vi "lab3.vi"() -> ()   [LabVIEW 2019]
uses:
  <vilib>/imath/engines/lvmath2/RunTimeEngine/BuiltInFunctions/iir_elliptic/NIMS_[2o]_iir_elliptic(I32,DBL2,V,Str).vi
  <vilib>/imath/engines/lvmath2/RunTimeEngine/ErrorHandling/NIMS_Create Error From Enums.vi
  <vilib>/imath/engines/lvmath/Plug In/Control Design/BuiltInFunctions/tf/NIMS_CD_tf(num,den,Ts).vi
  <vilib>/imath/engines/lvmath2/RunTimeEngine/BuiltInFunctions/iir_elliptic/NIMS_[3o]_iir_elliptic(I32,DBL2,V,Str).vi
  <vilib>/imath/engines/lvmath/Plug In/Control Design/BuiltInFunctions/zpk/NIMS_CD_zpk(zeros,poles,k,Ts).vi
  <vilib>/imathl/engines/lvmath/Functions/Error Handling/Create Error.vi
  <vilib>/imath/engines/lvmath2/RunTimeEngine/BuiltInFunctions/iir_elliptic/NIMS_[4o]_iir_elliptic(I32,DBL2,V,Str).vi
  <vilib>/imath/engines/lvmath/Plug In/Control Design/BuiltInFunctions/ss/NIMS_CD_ss(A,B,C,D).vi
  <vilib>/imath/engines/lvmath2/RunTimeEngine/NodeEndStatement/NIMS_NodeEndStatement_Output.vi
  <instcachedir>/0/NIMS_NodeEndStatement_Output_53EC0D466D134D7ABD903AC30B43404B.lvgen/NIMS_NodeEndStatement_Output_53EC0D466D134D7ABD903AC30B43404B_011.vi
  <instcachedir>/0/NIMS_NodeEndStatement_Output_53EC0D466D134D7ABD903AC30B43404B.lvgen/NIMS_NodeEndStatement_Output_53EC0D466D134D7ABD903AC30B43404B_010.vi
  <instcachedir>/0/NIMS_NodeEndStatement_Output_53EC0D466D134D7ABD903AC30B43404B.lvgen/NIMS_NodeEndStatement_Output_53EC0D466D134D7ABD903AC30B43404B_009.vi
  <vilib>/imath/engines/lvmath2/RunTimeEngine/ErrorHandling/NIMS_Finalize Error.vi
  <vilib>/addons/Control Design/_Time Response Analysis/Time Response.llb/Time Response subVI/cd_Step Response (State-Space).vi
  <vilib>/addons/Control Design/_Frequency Response Analysis/Frequency Response.llb/Frequency Response subVI/cd_Bode (State Space).vi
  <vilib>/addons/Control Design/_Utility/Model Viewer.llb/Model Viewer SubVI/cd_Draw State-Space Equation (SS).vi
  <vilib>/addons/Control Design/_Frequency Response Analysis/Frequency Response.llb/Frequency Response subVI/cd_Bode (Zero-Pole-Gain).vi
  <vilib>/addons/Control Design/_Time Response Analysis/Time Response.llb/Time Response subVI/cd_Step Response (Zero-Pole-Gain).vi
  <vilib>/addons/Control Design/_Utility/Model Viewer.llb/Model Viewer SubVI/cd_Draw Zero-Pole-Gain Equation (ZPK).vi
  <vilib>/addons/Control Design/_Frequency Response Analysis/Frequency Response.llb/Frequency Response subVI/cd_Bode (Transfer Function).vi
  <vilib>/addons/Control Design/_Time Response Analysis/Time Response.llb/Time Response subVI/cd_Step Response (Transfer Function).vi
  <vilib>/addons/Control Design/_Utility/Model Viewer.llb/Model Viewer SubVI/cd_Draw Transfer Function Equation (TF).vi
  <vilib>/addons/Control Design/_Utility/NI_CD_Model Viewer.lvlib
  <vilib>/addons/Control Design/_Time Response Analysis/NI_CD_Time Response.lvlib
  <vilib>/addons/Control Design/_Frequency Response Analysis/NI_CD_Frequency Response.lvlib
panel:
  out "ФЧХ":cluster{"time":dbl[], dbl[]}[](graph)
  out "Нули, полюса и коэффициент усиления (zpk)":picture
  out "Реакция на ступенчатое воздействие":cluster{"time":dbl[], dbl[]}[](graph)=[{"time"=[0.0, 0.01, 0.02, 0.03, 0.04, 0.05, 0.06, 0.07, 0.08, 0.09, 0.1, 0.11, 0.12, 0.13, 0.14, 0.15, 0.16, 0.17, 0.18, 0.19, 0.2, 0.21, 0.22, 0.23, 0.24, 0.25, 0.26, 0.27, 0.28, 0.29, 0.3, 0.31, 0.32, 0.33, 0.34, 0.35000000000000003, 0.36, 0.37, 0.38, 0.39, 0.4, 0.41000000000000003, 0.42, 0.43, 0.44, 0.45, 0.46, 0.47000000000000003, 0.48, 0.49, 0.5, 0.51, 0.52, 0.53, 0.54, 0.55, 0.56, 0.5700000000000001, 0.58, 0.59, 0.6, 0.61, 0.62, 0.63, 0.64, 0.65, 0.66, 0.67, 0.68, 0.6900000000000001, 0.7000000000000001, 0.71, 0.72, 0.73, 0.74, 0.75, 0.76, 0.77, 0.78, 0.79, 0.8, 0.81, 0.8200000000000001, 0.8300000000000001, 0.84, 0.85, 0.86, 0.87, 0.88, 0.89, 0.9, 0.91, 0.92, 0.93, 0.9400000000000001, 0.9500000000000001, 0.96, 0.97, 0.98, 0.99, 1.0], [0.0, 3.6082865061234616e-06, 1.1407278521072656e-05, 2.9529784958030634e-05, 6.642330456811847e-05, 0.00013503170249437238, 0.0002548548609154596, 0.0004541695796313746, 0.0007725569985214442, 0.0012637784461943145, 0.0019989621543555023, 0.003069999296471257, 0.004592993460926125, 0.006711559663559145, 0.009599726404238182, 0.013464158128184637, 0.018545388338242815, 0.025117739083195107, 0.03348760461422225, 0.04398979952247976, 0.05698171784936523, 0.07283512155630463, 0.09192547485599553, 0.11461886387244882, 0.14125668546765777, 0.17213844925750407, 0.20750320518044707, 0.2475102759907256, 0.29222012880100523, 0.34157635049365703, 0.3953897864575091, 0.4533259492913405, 0.5148967939113728, 0.579457880307616, 0.6462118005760611, 0.7142185322522965, 0.7824130992479892, 0.8496305834265399, 0.9146381473654828, 0.9761733198830131, 1.0329873819716318, 1.083892296189833, 1.1278092731232305, 1.1638167900206793, 1.191195693197778, 1.2094689478589153, 1.2184336620214729, 1.2181832139346669, 1.2091176555606453, 1.191941040408115, 1.1676449153653718, 1.1374778975653794, 1.1029019953315176, 1.0655370872304384, 1.0270957013066055, 0.9893108920932084, 0.9538605515110161, 0.9222918708899738, 0.8959498617110293, 0.8759138185733986, 0.8629453575615864, 0.8574511882916371, 0.8594630943828092, 0.8686367349695323, 0.8842698822165649, 0.9053396306961685, 0.9305570161479116, 0.9584364302320009, 0.987376281517763, 1.0157465941619432, 1.041978709252556, 1.0646520019267478, 1.0825725766873904, 1.0948392620397485, 1.1008928822866797, 1.1005457078265957, 1.0939891258287846, 1.0817788649680364, 1.0647984729633668, 1.0442030983895345, 1.0213468811312547, 0.9976983250429551, 0.9747488376536154, 0.9539201158763563, 0.9364761935847676, 0.9234457298339228, 0.9155595125950468, 0.9132072149517516, 0.9164162242253882, 0.9248539457574722, 0.9378534532892434, 0.9544608181330321, 0.9735010039080574, 0.993657960958816, 1.0135635844875825, 1.031889581311644, 1.0474360710593627, 1.0592109474021638, 1.0664946358591876, 1.0688858688517833, 1.0663253920793205]}, {"time"=[0.0, 0.01, 0.02, 0.03, 0.04, 0.05, 0.06, 0.07, 0.08, 0.09, 0.1, 0.11, 0.12, 0.13, 0.14, 0.15, 0.16, 0.17, 0.18, 0.19, 0.2, 0.21, 0.22, 0.23, 0.24, 0.25, 0.26, 0.27, 0.28, 0.29, 0.3, 0.31, 0.32, 0.33, 0.34, 0.35000000000000003, 0.36, 0.37, 0.38, 0.39, 0.4, 0.41000000000000003, 0.42, 0.43, 0.44, 0.45, 0.46, 0.47000000000000003, 0.48, 0.49, 0.5, 0.51, 0.52, 0.53, 0.54, 0.55, 0.56, 0.5700000000000001, 0.58, 0.59, 0.6, 0.61, 0.62, 0.63, 0.64, 0.65, 0.66, 0.67, 0.68, 0.6900000000000001, 0.7000000000000001, 0.71, 0.72, 0.73, 0.74, 0.75, 0.76, 0.77, 0.78, 0.79, 0.8, 0.81, 0.8200000000000001, 0.8300000000000001, 0.84, 0.85, 0.86, 0.87, 0.88, 0.89, 0.9, 0.91, 0.92, 0.93, 0.9400000000000001, 0.9500000000000001, 0.96, 0.97, 0.98, 0.99, 1.0], [0.0, 3.470187299156327e-24, 4.370315472509466e-19, 4.1169111270240676e-16, 5.210188934862779e-14, 2.1899713849440105e-12, 4.575063221464954e-11, 5.889795375843283e-10, 5.3120774653900036e-09, 3.6459470569347496e-08, 2.0148664582515347e-07, 9.333272030028442e-07, 3.7329029137926227e-06, 1.318377810255631e-05, 4.183832114899826e-05, 0.0001209538404944732, 0.0003220794631304584, 0.0007970612883164312, 0.0018466944730003332, 0.004030049956819416, 0.008325892189246425, 0.01635250951538534, 0.030640405862485856, 0.05493172544291945, 0.09445031608239979, 0.1560485866245648, 0.24809669666017425, 0.3799450479108828, 0.5607754249182307, 0.7976752704342736, 1.0928398313881935, 1.4399414652125764, 1.8199095283479387, 2.1966301852362657, 2.513377774887346, 2.691082392927966, 2.629756773270378, 2.21446944184742, 1.3270760315781527, -0.13556722182377876, -2.237028744662703, -4.971683130331221, -8.232840858682685, -11.783016865401411, -15.23221602666917, -18.031185810915638, -19.486900478300274, -18.80676233700509, -15.175867229116543, -7.868053910812445, 3.6135861075778477, 19.37719056120255, 38.98065461394668, 61.291451382972795, 84.3956776487094, 105.58624310660353, 121.45826630541379, 128.133154180371, 121.62109073135274, 98.31495878574687, 55.58807605641808, -7.554590054202641, -89.84417809684068, -187.22531097718198, -292.544421407455, -395.54999630659484, -483.29149855805167, -540.9740315375597, -553.2807607695211, -506.1169572969922, -388.66286688642197, -195.5542659933755, 71.05180937394306, 399.8133653942581, 769.2472751038177, 1147.7695869617626, 1494.964199240123, 1764.2124487935123, 1906.6779603818077, 1876.473128629441, 1636.6506663522107, 1165.4855238236921, 462.3623712467906, -447.5138870028618, -1510.3897508261405, -2643.9518692415513, -3740.59494476686, -4674.256253302845, -5310.7415579048575, -5521.043344830305, -5196.70660317422, -4265.87895532752, -2708.345578261108, -567.6497452353658, 2041.614977035666, 4933.05032787471, 7855.507889231544, 10508.562187339905, 12566.165875094744, 13707.286443472845, 13651.33328742056]}, {"time"=[0.0, 0.01, 0.02, 0.03, 0.04, 0.05, 0.06, 0.07, 0.08, 0.09, 0.1, 0.11, 0.12, 0.13, 0.14, 0.15, 0.16, 0.17, 0.18, 0.19, 0.2, 0.21, 0.22, 0.23, 0.24, 0.25, 0.26, 0.27, 0.28, 0.29, 0.3, 0.31, 0.32, 0.33, 0.34, 0.35000000000000003, 0.36, 0.37, 0.38, 0.39, 0.4, 0.41000000000000003, 0.42, 0.43, 0.44, 0.45, 0.46, 0.47000000000000003, 0.48, 0.49, 0.5, 0.51, 0.52, 0.53, 0.54, 0.55, 0.56, 0.5700000000000001, 0.58, 0.59, 0.6, 0.61, 0.62, 0.63, 0.64, 0.65, 0.66, 0.67, 0.68, 0.6900000000000001, 0.7000000000000001, 0.71, 0.72, 0.73, 0.74, 0.75, 0.76, 0.77, 0.78, 0.79, 0.8, 0.81, 0.8200000000000001, 0.8300000000000001, 0.84, 0.85, 0.86, 0.87, 0.88, 0.89, 0.9, 0.91, 0.92, 0.93, 0.9400000000000001, 0.9500000000000001, 0.96, 0.97, 0.98, 0.99, 1.0], [0.0, 3.470187299156327e-24, 4.370315472509466e-19, 4.116911127024068e-16, 5.2101889348627795e-14, 2.1899713849440113e-12, 4.5750632214649543e-11, 5.889795375843285e-10, 5.312077465390007e-09, 3.6459470569347516e-08, 2.0148664582515358e-07, 9.333272030028448e-07, 3.7329029137926265e-06, 1.3183778102556327e-05, 4.183832114899831e-05, 0.0001209538404944734, 0.00032207946313045897, 0.0007970612883164327, 0.0018466944730003369, 0.004030049956819425, 0.008325892189246445, 0.01635250951538538, 0.030640405862485946, 0.05493172544291962, 0.09445031608240011, 0.15604858662456542, 0.2480966966601753, 0.37994504791088457, 0.5607754249182335, 0.7976752704342779, 1.0928398313882002, 1.4399414652125857, 1.819909528347952, 2.1966301852362835, 2.513377774887368, 2.6910823929279917, 2.6297567732704055, 2.214469441847446, 1.3270760315781733, -0.13556722182377134, -2.237028744662715, -4.97168313033127, -8.232840858682778, -11.783016865401544, -15.232216026669352, -18.031185810915854, -19.486900478300498, -18.806762337005285, -15.175867229116648, -7.868053910812385, 3.6135861075781364, 19.37719056120318, 38.980654613947635, 61.29145138297406, 84.39567764871087, 105.58624310660507, 121.45826630541507, 128.13315418037155, 121.62109073135215, 98.3149587857447, 55.588076056414025, -7.554590054208546, -89.84417809684794, -187.2253109771894, -292.54442140746096, -395.54999630659665, -483.29149855804627, -540.974031537543, -553.2807607694906, -506.1169572969455, -388.6628668863589, -195.55426599329905, 71.05180937402588, 399.81336539433596, 769.2472751038736, 1147.7695869617764, 1494.9641992400684, 1764.212448793367, 1906.6779603815507, 1876.4731286290598, 1636.6506663517073, 1165.4855238230878, 462.36237124613353, -447.5138870034998, -1510.3897508266582, -2643.951869241824, -3740.5949447667454, -4674.256253302201, -5310.741557903557, -5521.043344828255, -5196.706603171397, -4265.878955323986, -2708.345578257037, -567.6497452310668, 2041.6149770397442, 4933.0503278779815, 7855.507889233315, 10508.562187339407, 12566.165875091217, 13707.28644346561, 13651.333287409152]}]
  out "Разница АЧХ, реализованных различным способом":cluster{"time":dbl[], dbl[]}[](graph)
  out "АЧХ":cluster{"time":dbl[], dbl[]}[](graph)
  out "Разница реакций на ступенчатое воздействие":cluster{"time":dbl[], dbl[]}[](graph)=[{"time"=[0.0, 0.01, 0.02, 0.03, 0.04, 0.05, 0.06, 0.07, 0.08, 0.09, 0.1, 0.11, 0.12, 0.13, 0.14, 0.15, 0.16, 0.17, 0.18, 0.19, 0.2, 0.21, 0.22, 0.23, 0.24, 0.25, 0.26, 0.27, 0.28, 0.29, 0.3, 0.31, 0.32, 0.33, 0.34, 0.35000000000000003, 0.36, 0.37, 0.38, 0.39, 0.4, 0.41000000000000003, 0.42, 0.43, 0.44, 0.45, 0.46, 0.47000000000000003, 0.48, 0.49, 0.5, 0.51, 0.52, 0.53, 0.54, 0.55, 0.56, 0.5700000000000001, 0.58, 0.59, 0.6, 0.61, 0.62, 0.63, 0.64, 0.65, 0.66, 0.67, 0.68, 0.6900000000000001, 0.7000000000000001, 0.71, 0.72, 0.73, 0.74, 0.75, 0.76, 0.77, 0.78, 0.79, 0.8, 0.81, 0.8200000000000001, 0.8300000000000001, 0.84, 0.85, 0.86, 0.87, 0.88, 0.89, 0.9, 0.91, 0.92, 0.93, 0.9400000000000001, 0.9500000000000001, 0.96, 0.97, 0.98, 0.99, 1.0], [0.0, 3.6082865061234616e-06, 1.140727852107222e-05, 2.9529784957618942e-05, 6.642330451601658e-05, 0.000135031700304401, 0.00025485481516482735, 0.00045416899065183706, 0.0007725516864439788, 0.0012637419867237451, 0.001998760667709677, 0.0030690659692682544, 0.004589260558012332, 0.006698375885456589, 0.009557888083089184, 0.013343204287690164, 0.018223308875112355, 0.024320677794878676, 0.03164091014122191, 0.039959749565660334, 0.048655825660118786, 0.05648261204091925, 0.061285068993509585, 0.059687138429529205, 0.04680636938525766, 0.016089862632938656, -0.04059349147972824, -0.13243477192015898, -0.2685552961172283, -0.45609891994062085, -0.6974500449306911, -0.9866155159212452, -1.3050127344365792, -1.6171723049286675, -1.8671659743113067, -1.9768638606756952, -1.8473436740224163, -1.3648388584209061, -0.41243788421269056, 1.1117405417067845, 3.2700161266343466, 6.055575426521103, 9.360650131806008, 12.946833655422223, 16.42341171986713, 19.24065475877477, 20.70533414032197, 20.02494555093995, 16.384984884677294, 9.0599949512205, -2.4459411922127643, -18.2397126636378, -37.87775261861612, -60.22591429574362, -83.36858194740427, -104.59693221451185, -120.50440575390405, -127.21086230948157, -120.72514086964112, -97.4390449671713, -54.72513069885244, 8.412041242500184, 90.70364119123074, 188.09394771215892, 293.42869128967754, 396.45533593729283, 484.2220555741942, 541.9324679677751, 554.2681370510084, 507.13270389110744, 389.70484559561146, 196.61891799522581, -69.96923679733848, -398.71852613229623, -768.1463822215869, -1146.66904125395, -1493.8702101142396, -1763.130669928399, -1905.6131619085875, -1875.4289255306703, -1635.629319470576, -1164.487825498045, -461.3876224084799, 448.4678071193762, 1511.3262270202429, 2644.875314971658, 3741.5105042793402, 4675.169460517152, 5311.657974127782, 5521.968198774012, 5197.6444566246855, 4266.833416142119, 2709.319079260945, 568.6434031920256, -2040.6014134552565, -4932.01843829667, -7854.460453162255, -10507.502976392005, -12565.099380455358, -13706.217557596758, -13650.266962017073]}, {"time"=[0.0, 0.01, 0.02, 0.03, 0.04, 0.05, 0.06, 0.07, 0.08, 0.09, 0.1, 0.11, 0.12, 0.13, 0.14, 0.15, 0.16, 0.17, 0.18, 0.19, 0.2, 0.21, 0.22, 0.23, 0.24, 0.25, 0.26, 0.27, 0.28, 0.29, 0.3, 0.31, 0.32, 0.33, 0.34, 0.35000000000000003, 0.36, 0.37, 0.38, 0.39, 0.4, 0.41000000000000003, 0.42, 0.43, 0.44, 0.45, 0.46, 0.47000000000000003, 0.48, 0.49, 0.5, 0.51, 0.52, 0.53, 0.54, 0.55, 0.56, 0.5700000000000001, 0.58, 0.59, 0.6, 0.61, 0.62, 0.63, 0.64, 0.65, 0.66, 0.67, 0.68, 0.6900000000000001, 0.7000000000000001, 0.71, 0.72, 0.73, 0.74, 0.75, 0.76, 0.77, 0.78, 0.79, 0.8, 0.81, 0.8200000000000001, 0.8300000000000001, 0.84, 0.85, 0.86, 0.87, 0.88, 0.89, 0.9, 0.91, 0.92, 0.93, 0.9400000000000001, 0.9500000000000001, 0.96, 0.97, 0.98, 0.99, 1.0], [0.0, 3.6082865061234616e-06, 1.140727852107222e-05, 2.9529784957618942e-05, 6.642330451601658e-05, 0.000135031700304401, 0.00025485481516482735, 0.00045416899065183706, 0.0007725516864439788, 0.0012637419867237451, 0.001998760667709677, 0.0030690659692682544, 0.004589260558012332, 0.006698375885456589, 0.009557888083089184, 0.013343204287690164, 0.018223308875112358, 0.024320677794878676, 0.03164091014122191, 0.03995974956566034, 0.04865582566011881, 0.05648261204091929, 0.061285068993509675, 0.05968713842952937, 0.04680636938525798, 0.016089862632939267, -0.040593491479727184, -0.1324347719201572, -0.2685552961172255, -0.4560989199406165, -0.6974500449306844, -0.9866155159212359, -1.3050127344365658, -1.6171723049286497, -1.867165974311285, -1.9768638606756694, -1.8473436740223887, -1.36483885842088, -0.4124378842126699, 1.1117405417067918, 3.270016126634335, 6.055575426521054, 9.360650131805915, 12.94683365542209, 16.423411719866948, 19.240654758774554, 20.705334140321746, 20.024945550939755, 16.384984884677188, 9.05999495122056, -2.4459411922124756, -18.23971266363717, -37.87775261861517, -60.225914295742356, -83.36858194740279, -104.59693221451032, -120.50440575390277, -127.21086230948103, -120.7251408696417, -97.43904496717347, -54.725130698856496, 8.412041242494277, 90.70364119122348, 188.0939477121515, 293.4286912896716, 396.455335937291, 484.2220555741996, 541.9324679677917, 554.2681370510388, 507.13270389115416, 389.7048455956745, 196.61891799530227, -69.96923679725566, -398.71852613221836, -768.1463822215311, -1146.669041253936, -1493.8702101142942, -1763.1306699285442, -1905.6131619088444, -1875.4289255310514, -1635.6293194710795, -1164.4878254986493, -461.38762240913695, 448.46780711873816, 1511.3262270197251, 2644.8753149713853, 3741.510504279455, 4675.169460517796, 5311.6579741290825, 5521.968198776062, 5197.644456627509, 4266.833416145653, 2709.319079265016, 568.6434031963246, -2040.6014134511784, -4932.0184382933985, -7854.460453160485, -10507.502976392503, -12565.099380458885, -13706.217557603994, -13650.266962028481]}]
  out "Передаточная функция":picture
  out "Модель в пространстве состояний":picture
  in  "dbp":dbl=0.05
  in  "n":dbl=5.0
  in  "dbs":dbl=120.0
  in  "w":dbl=5.0
  in  "Time Range":cluster{"t0":dbl, "dt":dbl, "tf":dbl}={"t0"=0.0, "dt"=0.01, "tf"=1.0}
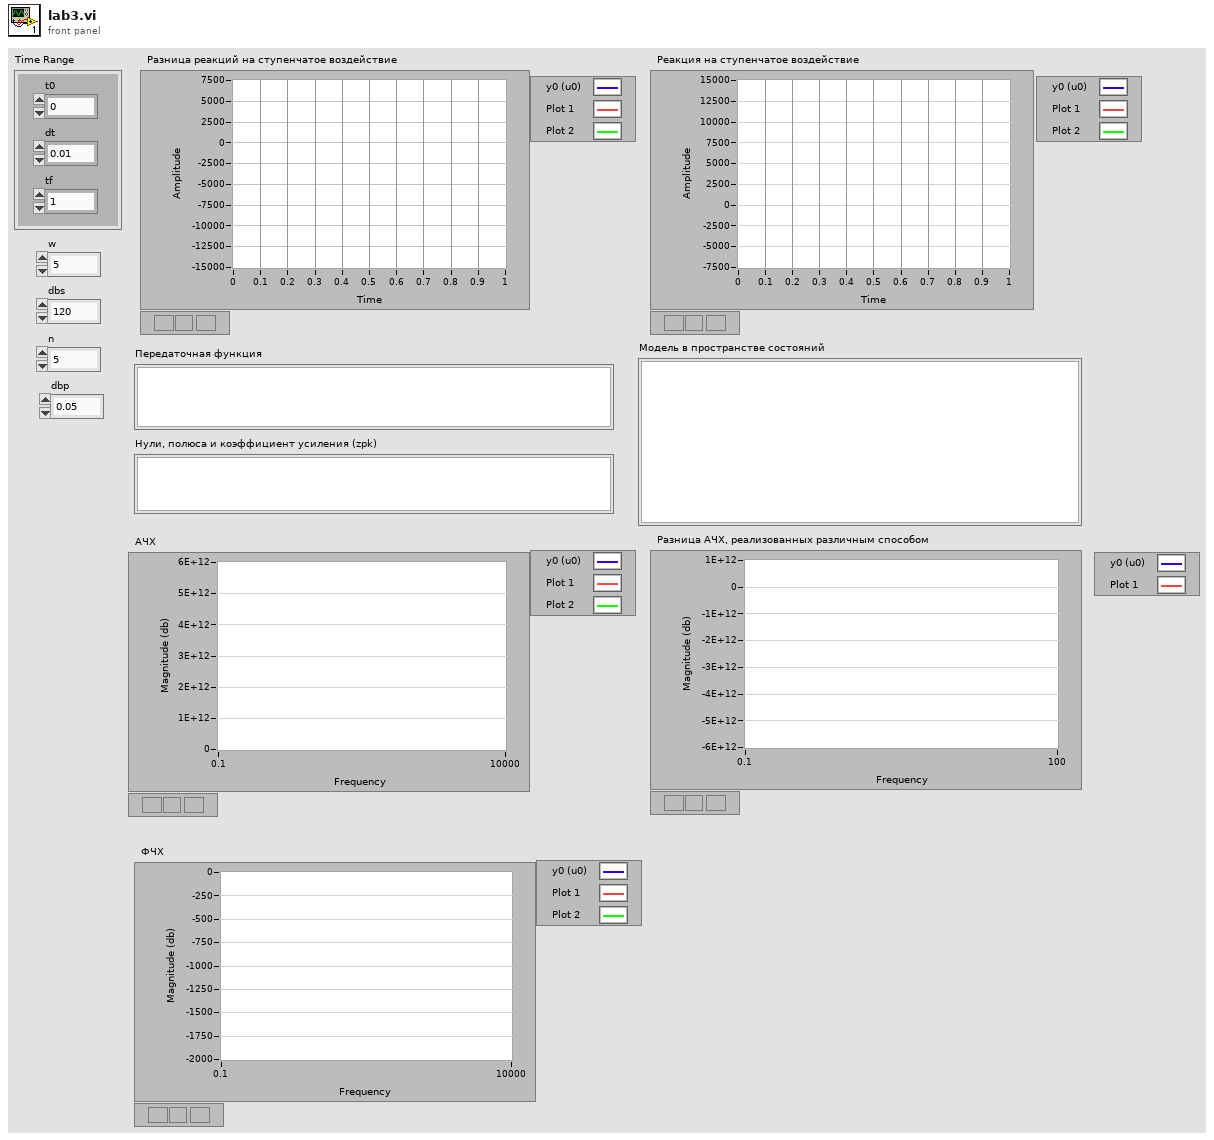
[diagram p1: front panel]
types:
  T1 = typedef "NI_LinSys_Model Typedefs.lvlib/CD Transfer Function Model (MIMO).ctl" = cluster{"properties":T2, "transfer function(s)":T3[][]}
  T2 = typedef "NI_LinSys_Model Typedefs.lvlib/CD General Elements.ctl" = cluster{"Model name":string, "Input names":string[], "Output names":string[], "Input Delays":dbl[], "Output Delays":dbl[], "Sampling Time":dbl, "Notes":string}
  T3 = typedef "NI_LinSys_Model Typedefs.lvlib/CD Transfer Function Model (SISO).ctl" = cluster{"Numerator":dbl[], "Denominator":dbl[], "delay":dbl}
  T4 = typedef "NI_LinSys_Model Typedefs.lvlib/CD Zero-Pole-Gain Model (MIMO).ctl" = cluster{"properties":T2, "zero-pole-gain(s)":T5[][]}
  T5 = typedef "NI_LinSys_Model Typedefs.lvlib/CD Zero-Pole-Gain Model (SISO).ctl" = cluster{"Gain":dbl, "Zeros":cdb[], "Poles":cdb[], "delay":dbl}
  T6 = typedef "NI_LinSys_Model Typedefs.lvlib/CD State Space Model (MIMO).ctl" = cluster{"properties":T2, "A":dbl[][], "B":dbl[][], "C":dbl[][], "D":dbl[][], "StateNames":string[], "Transport Delay":dbl[][]}
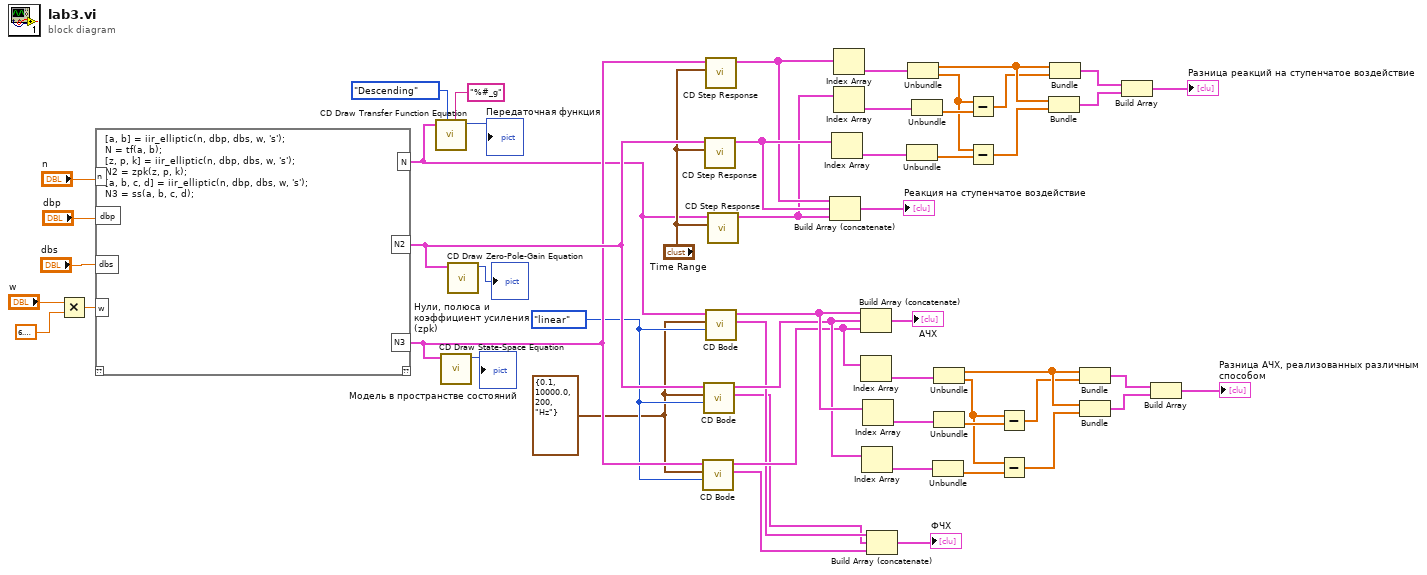
[diagram p0: block diagram]
diagram:
  w39 = enum16{"linear"}."linear"
  w38 = cluster{dbl, dbl, i32, enum16{"Hz"}} {0.1, 10000.0, 200, enum."Hz"} ("Frequency Range")
  n1 = Multiply(x="w", y=6.283185307179586) -> (x*y=w52:dbl)
  n2 = mathscript code="[a, b] = iir_elliptic(n, dbp, dbs, w, 's');\nN = tf(a, b);\n[z, p, k] = iir_elliptic(n, dbp, dbs, w, 's');\nN2 = zpk(z, p, k);\n[a, b, c, d] = iir_elliptic(n, dbp, dbs, w, 's');\nN3 = ss(a, b, c, d);"("n"="n", "dbp"="dbp", "dbs"="dbs", "w"=w52) -> ("N"=w40:T1, "N2"=w47:T4, "N3"=w41:T6)  [unwired: 1 in, 1 out]
  n3 = call-poly <vilib>:"CD Draw Transfer Function Equation.vi"("Format Coefficients"="%#_g", "Display Format"=enum16{"", "Ascending", "Descending"}."Descending", "Transfer Function Model"=w40) -> ("Equation"=→"Передаточная функция":picture)  [unwired: 6 in, 2 out]
  n4 = call-poly <vilib>:"CD Draw State-Space Equation.vi"("State-Space Model"=w41) -> ("Equation"=→"Модель в пространстве состояний":picture)  [unwired: 8 in, 2 out]
  n5 = call-poly <vilib>:"CD Draw Zero-Pole-Gain Equation.vi"("Zero-Pole-Gain Model"=w47) -> ("Equation"=→"Нули, полюса и коэффициент усиления (zpk)":picture)  [unwired: 8 in, 2 out]
  n6 = call-poly <vilib>:"CD Bode.vi"("Magnitude Scale"=w39, "Frequency Range"=w38, "State-Space Model"=w41) -> ("Bode Phase"=w1:cluster{"W":dbl[], "Magnitude":dbl[]}[], "Bode Magnitude"=w26:cluster{"W":dbl[], "Magnitude":dbl[]}[])  [unwired: 4 in, 3 out]
  n7 = call-poly <vilib>:"CD Bode.vi"("Magnitude Scale"=w39, "Frequency Range"=w38, "Zero-Pole-Gain Model"=w47) -> ("Bode Phase"=w2:cluster{"W":dbl[], "Magnitude":dbl[]}[], "Bode Magnitude"=w27:cluster{"W":dbl[], "Magnitude":dbl[]}[])  [unwired: 4 in, 3 out]
  n8 = call-poly <vilib>:"CD Step Response.vi"("Time Range"="Time Range", "Zero-Pole-Gain Model"=w47) -> ("Step Response Graph"=w7:cluster{"time":dbl[], dbl[]}[])  [unwired: 7 in, 2 out]
  n9 = call-poly <vilib>:"CD Step Response.vi"("Time Range"="Time Range", "State-Space Model"=w41) -> ("Step Response Graph"=w6:cluster{"time":dbl[], dbl[]}[])  [unwired: 6 in, 3 out]
  n10 = call-poly <vilib>:"CD Bode.vi"("Magnitude Scale"=w39, "Frequency Range"=w38, "Transfer Function Model"=w40) -> ("Bode Phase"=w3:cluster{"W":dbl[], "Magnitude":dbl[]}[], "Bode Magnitude"=w28:cluster{"W":dbl[], "Magnitude":dbl[]}[])  [unwired: 4 in, 3 out]
  n11 = call-poly <vilib>:"CD Step Response.vi"("Time Range"="Time Range", "Transfer Function Model"=w40) -> ("Step Response Graph"=w5:cluster{"time":dbl[], dbl[]}[])  [unwired: 7 in, 2 out]
  n12 = Build Array (concatenate)(w6, w7, w5) -> (→"Реакция на ступенчатое воздействие":cluster{"time":dbl[], dbl[]}[])
  n13 = Index Array(array=w7) -> (element=w35:cluster{"time":dbl[], dbl[]})  [unwired: 1 in]
  n14 = Index Array(array=w6) -> (element=w37:cluster{"time":dbl[], dbl[]})  [unwired: 1 in]
  n15 = Index Array(array=w5) -> (element=w36:cluster{"time":dbl[], dbl[]})  [unwired: 1 in]
  n16 = Build Array (concatenate)(w28, w27, w26) -> (→"АЧХ":cluster{"W":dbl[], "Magnitude":dbl[]}[])
  n17 = Index Array(array=w26) -> (element=w25:cluster{"W":dbl[], "Magnitude":dbl[]})  [unwired: 1 in]
  n18 = Index Array(array=w27) -> (element=w23:cluster{"W":dbl[], "Magnitude":dbl[]})  [unwired: 1 in]
  n19 = Index Array(array=w28) -> (element=w24:cluster{"W":dbl[], "Magnitude":dbl[]})  [unwired: 1 in]
  n20 = Build Array (concatenate)(w3, w2, w1) -> (→"ФЧХ":cluster{"W":dbl[], "Magnitude":dbl[]}[])
  n21 = Unbundle(w35) -> (w32:dbl[])  [unwired: 1 out]
  n22 = Unbundle(w37) -> ("time"=w34:dbl[], w31:dbl[])
  n23 = Unbundle(w36) -> (w33:dbl[])  [unwired: 1 out]
  n24 = Unbundle(w23) -> ("Magnitude"=w21:dbl[])  [unwired: 1 out]
  n25 = Unbundle(w25) -> ("W"=w20:dbl[], "Magnitude"=w8:dbl[])
  n26 = Unbundle(w24) -> ("Magnitude"=w22:dbl[])  [unwired: 1 out]
  n27 = Subtract(x=w31, y=w33) -> (x-y=w30:dbl[])
  n28 = Subtract(x=w31, y=w32) -> (x-y=w29:dbl[])
  n29 = Subtract(x=w8, y=w22) -> (x-y=w19:dbl[])
  n30 = Subtract(x=w8, y=w21) -> (x-y=w18:dbl[])
  n31 = Bundle("time"=w34, w29) -> (w16:cluster{"time":dbl[], dbl[]})  [unwired: 1 in]
  n32 = Bundle("time"=w34, w30) -> (w17:cluster{"time":dbl[], dbl[]})  [unwired: 1 in]
  n33 = Bundle("W"=w20, w19) -> (w15:cluster{"W":dbl[], dbl[]})  [unwired: 1 in]
  n34 = Bundle("W"=w20, w18) -> (w14:cluster{"W":dbl[], dbl[]})  [unwired: 1 in]
  n35 = Build Array(w17, w16) -> (→"Разница реакций на ступенчатое воздействие":cluster{"time":dbl[], dbl[]}[])
  n36 = Build Array(w15, w14) -> (→"Разница АЧХ, реализованных различным способом":cluster{"W":dbl[], dbl[]}[])
